vi "Read SS with Header.vi"(11 "Transpose Data Array":bool) -> (4 "Header String":string, 8 "Data Read":dbl[][](array[numeric]) format="%.2f", 15 "cancelled":bool)   [LabVIEW 2017]
doc: "This vi reads a 2D spreadsheet and a text header from a file. It is meant to work specifically with Write SS with Header.vi\n\nThe parser string is [CR, CR, DDD, CR, CR]."
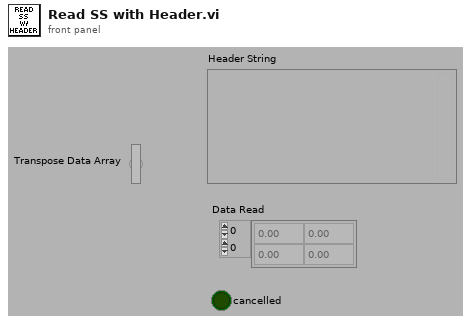
[diagram p1: front panel]
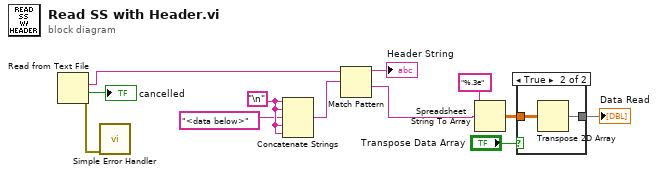
[diagram p0: block diagram]
diagram:
  w12 = "\n"
  n1 = Read from Text File() -> (text=w7:string, cancelled=→"cancelled":bool, error out=w9:errorcluster)  [unwired: 4 in, 1 out]
  n2 = call <vilib>:"Simple Error Handler.vi"("error in (no error)"=w9) -> ()  [unwired: 4 in, 5 out]
  n3 = Concatenate Strings(w12, w12, "<data below>", w12, w12) -> (w6:string)
  n4 = Match Pattern(string=w7, regular expression=w6) -> (before substring=→"Header String":string, after substring=w1:string)  [unwired: 1 in, 2 out]
  n5 = Spreadsheet String To Array(format string="%.3e", spreadsheet string=w1) -> (array=w5:dbl[][])  [unwired: 2 in]
  n6 = case shown="True" "Transpose Data Array" {
    tunnel: w5 -> [w13 w15]
    tunnel: [w13 w14] -> w2
    frame False {
    }
    frame True {
      n7 = Transpose 2D Array(2D array=w15) -> (transposed array=w14:dbl[][])
    }
  }
  "Data Read" <- w2
